vi "Shutdown.vi"(8 "error in (no error)":errorcluster, 11 "DMM in":refnum<class "DMM.lvclass">) -> (0 "error out":errorcluster, 3 "DMM out":refnum<class "DMM.lvclass">)   [LabVIEW 2018, in "DMM.lvlib" / "DMM.lvclass"]
uses:
  DMM.lvclass
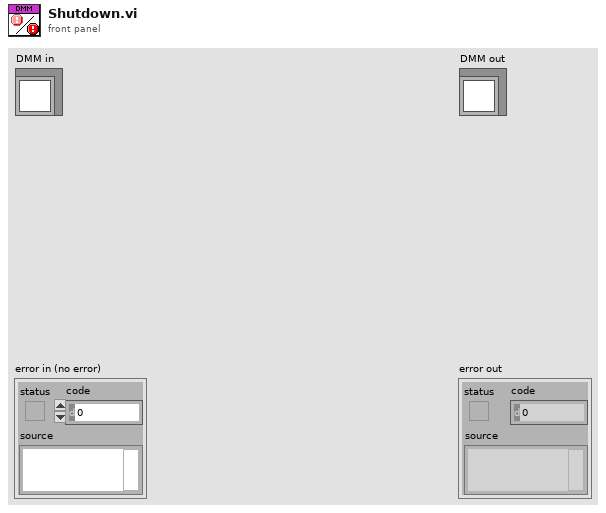
[diagram p1: front panel]
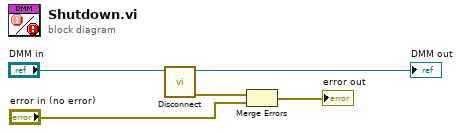
[diagram p0: block diagram]
diagram:
  n1 = call-dynamic "Disconnect.vi"("DMM in"="DMM in") -> ("error out"=w3:errorcluster, "DMM out"=→"DMM out":refnum<class "DMM.lvclass">)  [unwired: 9 in]
  n2 = Merge Errors(w3, "error in (no error)") -> (→"error out":errorcluster)
